vi "20-2.vi"() -> ()   [LabVIEW 2019, in "20.lvlib"]
uses:
  20.lvlib
panel:
  in  "Sample?":bool
  out "Lit":i16
  in  "Steps":i32
  out "Transformed Image":i16[][](graph)
  out "Initial Image":i16[][](graph)
  out "substring before match":string
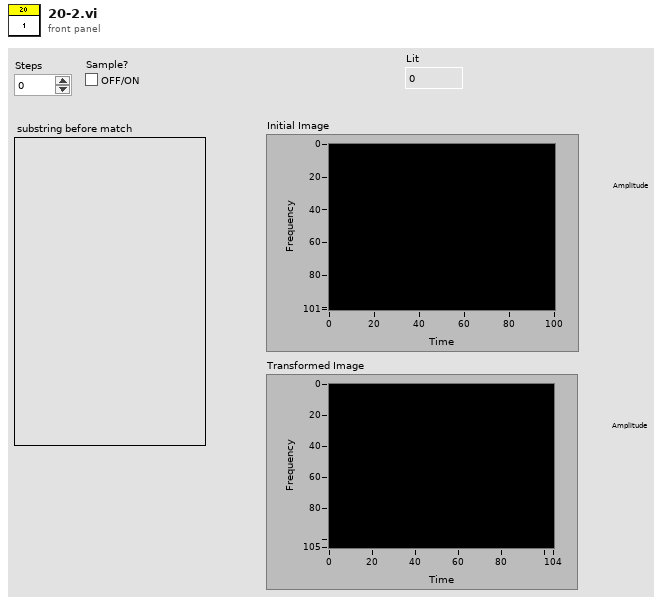
[diagram p1: front panel]
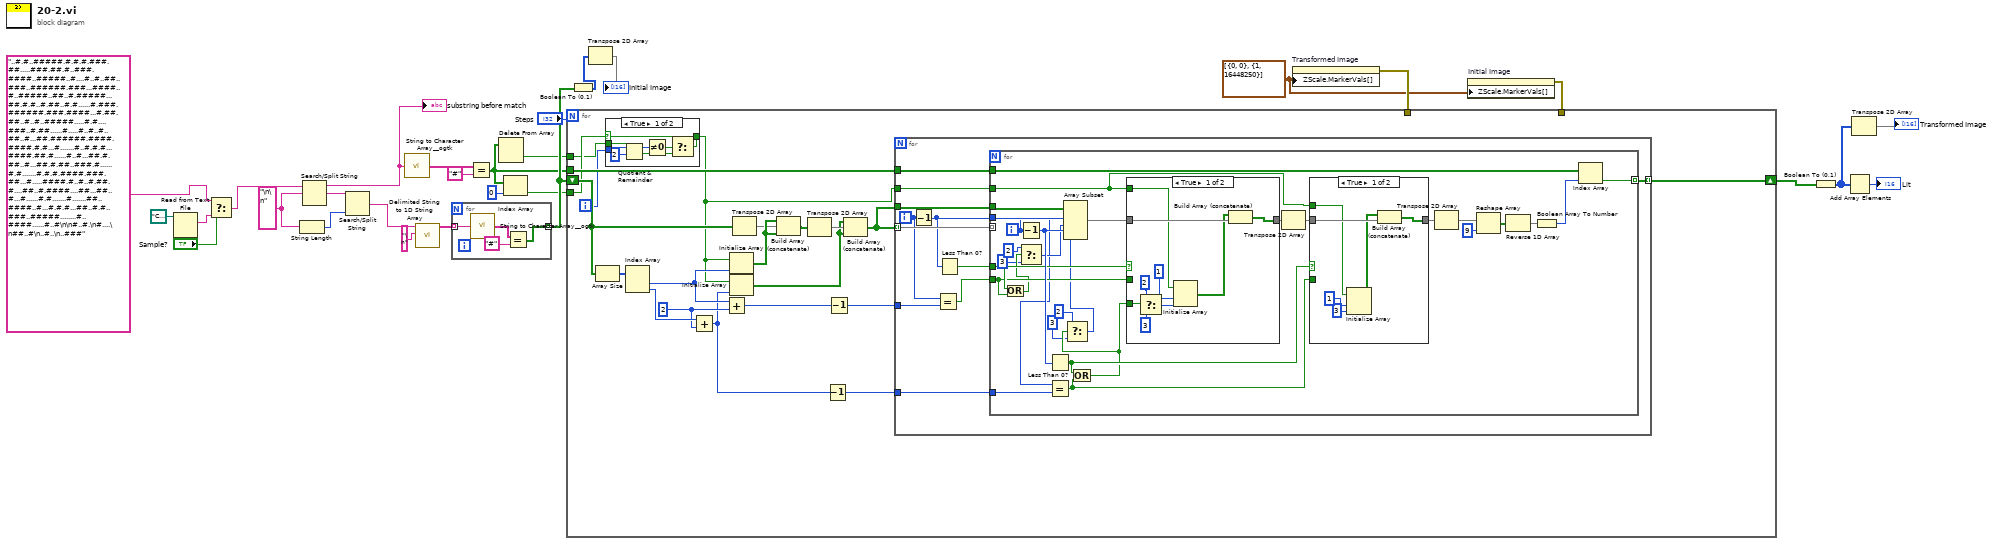
[diagram p0: block diagram]
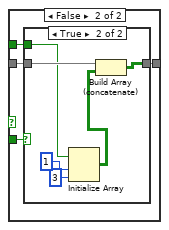
[diagram p2: hidden frame]
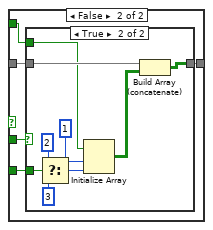
[diagram p4: hidden frame]
diagram:
  w17 = cluster{i16, u32}[] [{0, 0}, {1, 16448250}] ("Z Scale.Marker Values[]")
  w29 = "\n\n" ("search string/char (-)")
  n1 = Read from Text File(file (use dialog)=path "C:/Users/craig.walker/Documents/GitHub/lv2019-Advent-of-Code-2021/20/input.txt") -> (text=w13:string)  [unwired: 3 in, 3 out]
  n2 = Select(t="..#.#..#####.#.#.#.###.##.....###.##.#..###.####..#####..#....#..#..##..###..######.###...####..#..#####..##..#.#####...##.#.#..#.##..#.#......#.###.######.###.####...#.##.##..#..#..#####.....#.#....###..#.##......#.....#..#..#..##..#...##.######.####.####.#.#...#.......#..#.#.#...####.##.#......#..#...##.#.##..#...##.#.##..###.#......#.#.......#.#.#.####.###.##...#.....####.#..#..#.##.#....##..#.####....##...##..#...#......#.#.......#.......##..####..#...#.#.#...##..#.#..###..#####........#..####......#..#\n\n#..#.\n#....\n##..#\n..#..\n..###", s="Sample?", f=w13) -> (s? t:f=w11:string)
  n3 = String Length(string=w29) -> (length=w27:i32)
  n4 = Search/Split String(string=w11, search string/char (-)=w29) -> (substring before match=w23:string, match + rest of string=w28:string)  [unwired: 1 in, 1 out]
  "substring before match" <- w23
  n5 = Search/Split String(string=w28, offset (0)=w27) -> (match + rest of string=w26:string)  [unwired: 1 in, 2 out]
  n6 = call <userlib>:"String to Character Array__ogtk.vi"("Input String"=w23) -> ("Character Array"=w21:string[])
  n7 = call <vilib>:"Delimited String to 1D String Array.vi"("delimiter"="\n", "delimited string"=w26) -> ("string array"=w24:string[])  [unwired: 9 in]
  n8 = for {
    tunnel: w24 -> [w33] mode=indexing
    tunnel: [w30] -> w18 mode=indexing
    n9 = call <userlib>:"String to Character Array__ogtk.vi"("Input String"=w33) -> ("Character Array"=w31:string[])
    n10 = Equal?(x=w31, y="#") -> (x = y?=w30:bool[])
  }
  n11 = Equal?(x=w21, y="#") -> (x = y?=w6:bool[])
  n12 = Delete From Array(array=w6) -> (deleted portion=w5:bool)  [unwired: 2 in, 1 out]
  n13 = Index Array(array=w6, index=0) -> (element=w7:bool)
  n14 = Boolean To (0,1)(Boolean=w18) -> (0, 1=w15:i16[][])
  n15 = Transpose 2D Array(2D array=w15) -> (transposed array=→"Initial Image":i16[][])
  n16 = property on="Transformed Image" class="IntGraph (strict)"("ZScale.MarkerVals[]"=w17) -> (error out=w19:errorcluster)  [unwired: 2 in, 1 out]
  n17 = property on="Initial Image" class="IntGraph (strict)"("ZScale.MarkerVals[]"=w17) -> (error out=w16:errorcluster)  [unwired: 2 in, 1 out]
  n18 = for {
    N: "Steps" -> [_]
    tunnel: w6 -> [w48]
    shift-right: [w34] -> w2
    shift-left: w18 -> [w41]
    tunnel: w19 -> [_]
    tunnel: w16 -> [_]
    tunnel: w7 -> [w38]
    tunnel: w5 -> [w36]
    i -> [w37]
    w44 = 2 ("y")
    n19 = Array Size(array=w41) -> (size(s)=w54:i32[])
    n20 = case shown="True" w38 {
      selector: w38 -> [w138 w143]
      tunnel: w37 -> [w142 _]
      tunnel: [w136 w143] -> w35
      tunnel: w36 -> [w137 _]
      frame True {
        n21 = Quotient & Remainder(x=w142, y=2) -> (x-y*floor(x/y)=w140:i32)  [unwired: 1 out]
        n22 = Not Equal To 0?(x=w140) -> (x != 0?=w139:bool)
        n23 = Select(t=w138, s=w139, f=w137) -> (s? t:f=w136:bool)
      }
      frame False {
      }
    }
    n24 = Index Array(array=w54) -> (element #1=w45:i32, element #2=w47:i32)  [unwired: 2 in]
    n25 = Add(x=w47, y=w44) -> (x+y=w42:i32)
    n26 = Add(x=w45, y=w44) -> (x+y=w43:i32)
    n27 = Initialize Array(w35, w45) -> (w53:bool[])
    n28 = Initialize Array(w35, w42) -> (w46:bool[])
    n29 = Transpose 2D Array(2D array=w41) -> (transposed array=w49:bool[][])
    n30 = Build Array (concatenate)(w53, w49, w53) -> (w52:bool[][])
    n31 = Transpose 2D Array(2D array=w52) -> (transposed array=w51:bool[][])
    n32 = Decrement(x=w42) -> (x-1=w39:i32)
    n33 = Decrement(x=w43) -> (x-1=w40:i32)
    n34 = Build Array (concatenate)(w46, w51, w46) -> (w50:bool[][])
    n35 = for {
      tunnel: w50 -> [w65] mode=indexing
      tunnel: w50 -> [w64]
      tunnel: w48 -> [w63]
      tunnel: w40 -> [w61]
      tunnel: w39 -> [w60]
      tunnel: [w57] -> w34 mode=indexing
      tunnel: w35 -> [w55]
      i -> [w56]
      n36 = Decrement(x=w56) -> (x-1=w62:i32)
      n37 = Equal?(x=w56, y=w61) -> (x = y?=w58:bool)
      n38 = Less Than 0?(x=w62) -> (x < 0?=w59:bool)
      n39 = for {
        tunnel: w65 -> [_] mode=indexing
        tunnel: w64 -> [w94]
        tunnel: w63 -> [w90]
        tunnel: w62 -> [w93]
        tunnel: w60 -> [w87]
        tunnel: w59 -> [w81]
        tunnel: w58 -> [w80]
        tunnel: [w83] -> w57 mode=indexing
        tunnel: w55 -> [w66]
        i -> [w67]
        n40 = Or(x=w81, y=w80) -> (x .or. y?=w79:bool)
        n41 = Decrement(x=w67) -> (x-1=w88:i32)
        n42 = Select(t=2 ("length"), s=w79, f=3) -> (s? t:f=w78:i32)
        n43 = Less Than 0?(x=w88) -> (x < 0?=w85:bool)
        n44 = Equal?(x=w67, y=w87) -> (x = y?=w84:bool)
        n45 = Or(x=w85, y=w84) -> (x .or. y?=w76:bool)
        n46 = Select(t=2 ("length"), s=w76, f=3) -> (s? t:f=w73:i32)
        n47 = Array Subset(array=w94, index (row)=w93, length (row)=w78, index (col)=w88, length (col)=w73) -> (w72:bool[][])
        n48 = case shown="True" w81 {
          tunnel: w72 -> [w120 w125]
          tunnel: [w119 w124] -> w71
          tunnel: w76 -> [w114 w123]
          tunnel: w80 -> [_ w122]
          tunnel: w66 -> [w112 w121]
          frame True {
            n49 = Select(t=2, s=w114, f=3) -> (s? t:f=w115:i32)
            n50 = Initialize Array(w112, 1, w115) -> (w113:bool[][])
            n51 = Build Array (concatenate)(w113, w120) -> (w119:bool[][])
          }
          frame False {
            n52 = case shown="True" w122 {
              tunnel: w125 -> [w126 w135]
              tunnel: [w126 w134] -> w124
              tunnel: w123 -> [_ w130]
              tunnel: w121 -> [_ w133]
              frame False {
              }
              frame True {
                n53 = Select(t=2, s=w130, f=3) -> (s? t:f=w127:i32)
                n54 = Initialize Array(w133, 1, w127) -> (w132:bool[][])
                n55 = Build Array (concatenate)(w135, w132) -> (w134:bool[][])
              }
            }
          }
        }
        n56 = Transpose 2D Array(2D array=w71) -> (transposed array=w70:bool[][])
        n57 = case shown="True" w85 {
          tunnel: w70 -> [w100 w104]
          tunnel: [w99 w103] -> w86
          tunnel: w84 -> [_ w102]
          tunnel: w66 -> [w96 w101]
          frame True {
            n58 = Initialize Array(w96, 1, 3 ("dimension size")) -> (w95:bool[][])
            n59 = Build Array (concatenate)(w95, w100) -> (w99:bool[][])
          }
          frame False {
            n60 = case shown="True" w102 {
              tunnel: w104 -> [w105 w111]
              tunnel: [w105 w110] -> w103
              tunnel: w101 -> [_ w106]
              frame False {
              }
              frame True {
                n61 = Initialize Array(w106, 1, 3 ("dimension size")) -> (w107:bool[][])
                n62 = Build Array (concatenate)(w111, w107) -> (w110:bool[][])
              }
            }
          }
        }
        n63 = Transpose 2D Array(2D array=w86) -> (transposed array=w69:bool[][])
        n64 = Reshape Array(w69, 9 ("dimension size")) -> (w91:bool[])
        n65 = Reverse 1D Array(array=w91) -> (reversed array=w68:bool[])
        n66 = Boolean Array To Number(Boolean array=w68) -> (number=w89:u16)
        n67 = Index Array(array=w90, index=w89) -> (element=w83:bool)
      }
    }
  }
  n68 = Boolean To (0,1)(Boolean=w2) -> (0, 1=w4:i16[][])
  n69 = Add Array Elements(numeric array=w4) -> (sum=→"Lit":i16)
  n70 = Transpose 2D Array(2D array=w4) -> (transposed array=→"Transformed Image":i16[][])
